vi "#76_MAV_MSG_COMMAND_LONG_ENCODE.vi"(10 "packet_sequence_in":u8, 11 "COMMAND_LONG":T1={"self"={"system_id"=255, "component_id"=190}, "target_system"=1, "target_component"=1, "command (MAV_CMD)"=0, "confirmation"=0, "param1"=0.0, "param2"=0.0, "param3"=0.0, "param4"=0.0, "param5"=0.0, "param6"=0.0, "param7"=0.0}) -> (2 "packet_sequence_out":u8, 3 "mavlink_buffer_out":u8[](array[numeric]))   [LabVIEW 2023]
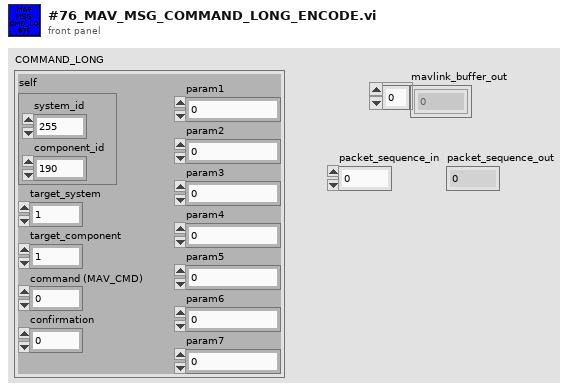
[diagram p1: front panel]
types:
  T1 = cluster{"self":cluster{"system_id":u8, "component_id":u8}, "target_system":u8, "target_component":u8, "command (MAV_CMD)":u16, "confirmation":u8, "param1":sgl, "param2":sgl, "param3":sgl, "param4":sgl, "param5":sgl, "param6":sgl, "param7":sgl}
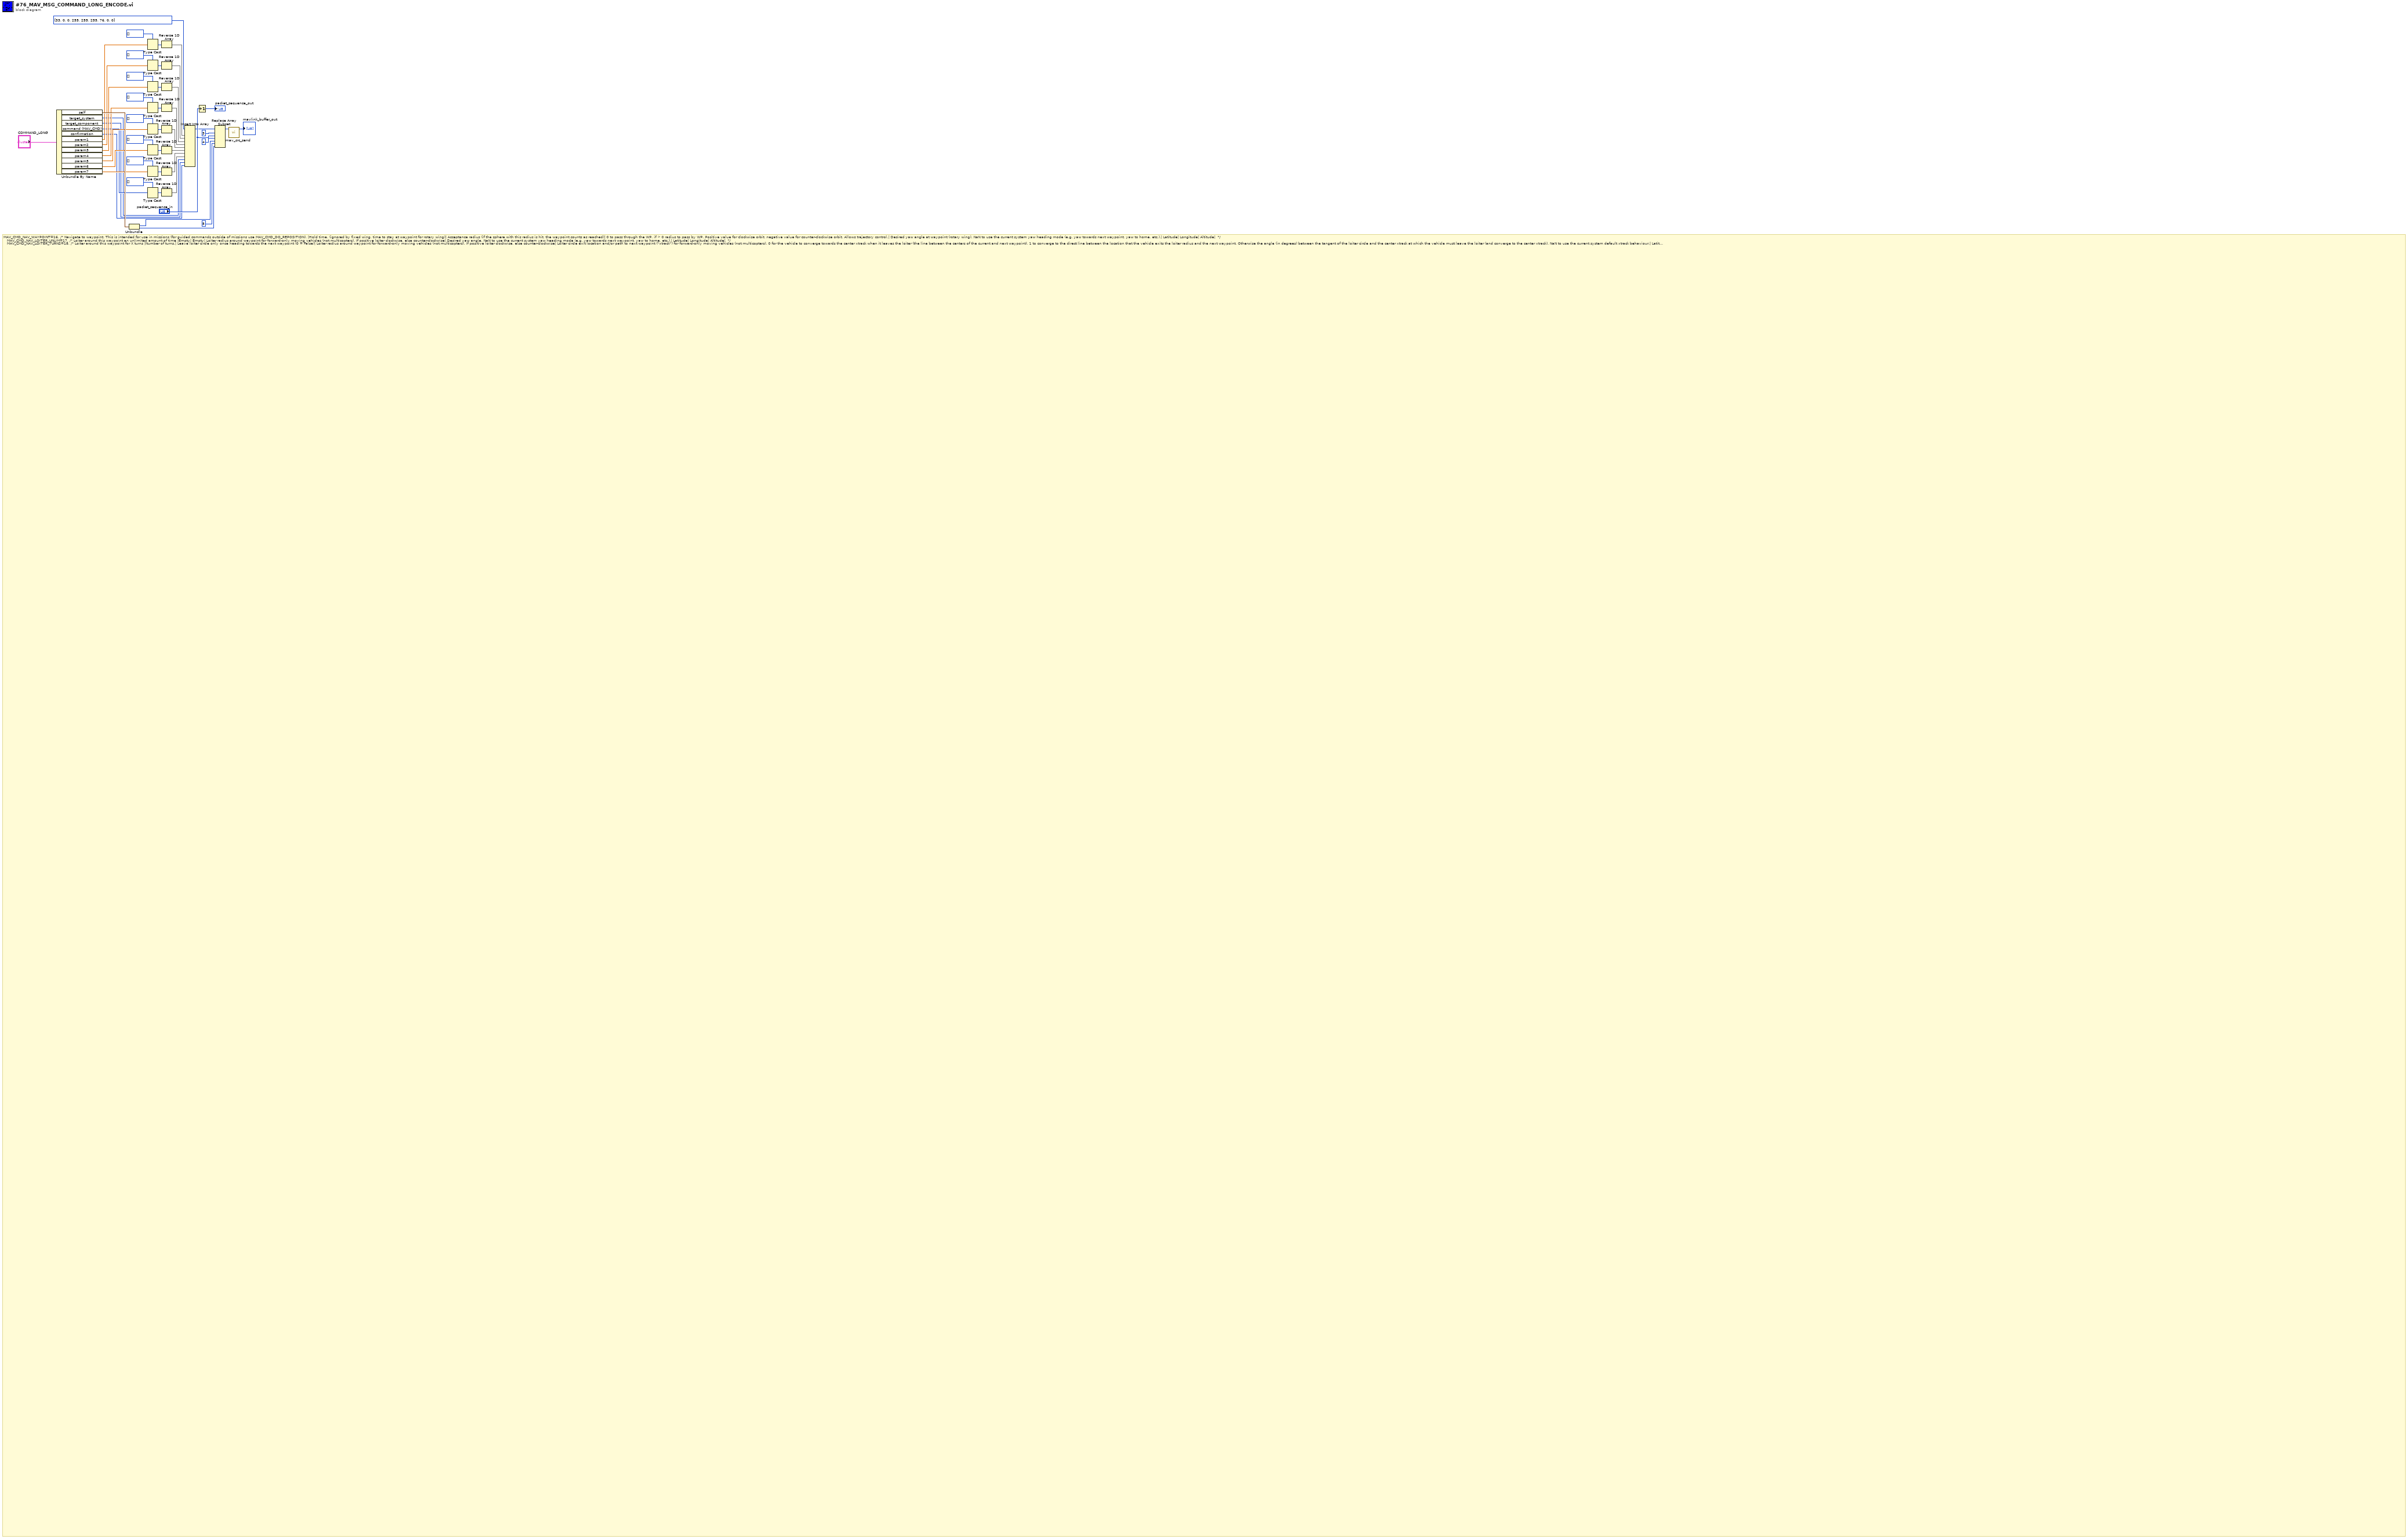
[diagram p0: block diagram]
diagram:
  # "MAV_CMD_NAV_WAYPOINT=16, /* Navigate to waypoint. This is intended for use in missions (for guided commands outside of missions use MAV_CMD_DO_REPOSITION). |Hold time. (ignored by fixed wing, time to stay at waypoint for rotary wing)| Acceptance radius (if the sphere with this radius is hit, the waypoint counts as reached)| 0 to pass through the WP, if > 0 radius to pass by WP. Positive value for clockwise orbit, negative value for counter-clockwise orbit. Allows trajectory control.| Desired yaw angle at waypoint (rotary wing). NaN to use the current system yaw heading mode (e.g. yaw towards next waypoint, yaw to home, etc.).| Latitude| Longitude| Altitude|  */\n   MAV_CMD_NAV_LOITER_UNLIM=17, /* Loiter around this waypoint an unlimited amount of time |Empty| Empty| Loiter radius around waypoint for forward-only moving vehicles (not multicopters). If positive loiter clockwise, else counter-clockwise| Desired yaw angle. NaN to use the current system yaw heading mode (e.g. yaw towards next waypoint, yaw to home, etc.).| Latitude| Longitude| Altitude|  */\n   MAV_CMD_NAV_LOITER_TURNS=18, /* Loiter around this waypoint for X turns |Number of turns.| Leave loiter circle only once heading towards the next waypoint (0 = False)| Loiter radius around waypoint for forward-only moving vehicles (not multicopters). If positive loiter clockwise, else counter-clockwise| Loiter circle exit location and/or path to next waypoint (\"xtrack\") for forward-only moving vehicles (not multicopters). 0 for the vehicle to converge towards the center xtrack when it leaves the loiter (the line between the centers of the current and next waypoint), 1 to converge to the direct line between the location that the vehicle exits the loiter radius and the next waypoint. Otherwise the angle (in degrees) between the tangent of the loiter circle and the center xtrack at which the vehicle must leave the loiter (and converge to the center xtrack). NaN to use the current system default xtrack behaviour.| Latitude| Longitude| Altitude|  */\n   MAV_CMD_NAV_LOITER_TIME=19, /* Loiter at the specified latitude, longitude and altitude for a certain amount of time. Multicopter vehicles stop at the point (within a vehicle-specific acceptance radius). Forward-only moving vehicles (e.g. fixed-wing) circle the point with the specified radius/direction. If the Heading Required parameter (2) is non-zero forward moving aircraft will only leave the loiter circle once heading towards the next waypoint. |Loiter time (only starts once Lat, Lon and Alt is reached).| Leave loiter circle only once heading towards the next waypoint (0 = False)| Loiter radius around waypoint for forward-only moving vehicles (not multicopters). If positive loiter clockwise, else counter-clockwise.| Loiter circle exit location and/or path to next waypoint (\"xtrack\") for forward-only moving vehicles (not multicopters). 0 for the vehicle to converge towards the center xtrack when it leaves the loiter (the line between the centers of the current and next waypoint), 1 to converge to the direct line between the location that the vehicle exits the loiter radius and the next waypoint. Otherwise the angle (in degrees) between the tangent of the loiter circle and the center xtrack at which the vehicle must leave the loiter (and converge to the center xtrack). NaN to use the current system default xtrack behaviour.| Latitude| Longitude| Altitude|  */\n   MAV_CMD_NAV_RETURN_TO_LAUNCH=20, /* Return to launch location |Empty| Empty| Empty| Empty| Empty| Empty| Empty|  */\n   MAV_CMD_NAV_LAND=21, /* Land at location. |Minimum target altitude if landing is aborted (0 = undefined/use system default).| Precision land mode.| Empty.| Desired yaw angle. NaN to use the current system yaw heading mode (e.g. yaw towards next waypoint, yaw to home, etc.).| Latitude.| Longitude.| Landing altitude (ground level in current frame).|  */\n   MAV_CMD_NAV_TAKEOFF=22, /* Takeoff from ground / hand. Vehicles that support multiple takeoff modes (e.g. VTOL quadplane) should take off using the currently configured mode. |Minimum pitch (if airspeed sensor present), desired pitch without sensor| Empty| Empty| Yaw angle (if magnetometer present), ignored without magnetometer. NaN to use the current system yaw heading mode (e.g. yaw towards next waypoint, yaw to home, etc.).| Latitude| Longitude| Altitude|  */\n   MAV_CMD_NAV_LAND_LOCAL=23, /* Land at local position (local frame only) |Landing target number (if available)| Maximum accepted offset from desired landing position - computed magnitude from spherical coordinates: d = sqrt(x^2 + y^2 + z^2), which gives the maximum accepted distance between the desired landing position and the position where the vehicle is about to land| Landing descend rate| Desired yaw angle| Y-axis position| X-axis position| Z-axis / ground level position|  */\n   MAV_CMD_NAV_TAKEOFF_LOCAL=24, /* Takeoff from local position (local frame only) |Minimum pitch (if airspeed sensor present), desired pitch without sensor| Empty| Takeoff ascend rate| Yaw angle (if magnetometer or another yaw estimation source present), ignored without one of these| Y-axis position| X-axis position| Z-axis position|  */\n   MAV_CMD_NAV_FOLLOW=25, /* Vehicle following, i.e. this waypoint represents the position of a moving vehicle |Following logic to use (e.g. loitering or sinusoidal following) - depends on specific autopilot implementation| Ground speed of vehicle to be followed| Radius around waypoint. If positive loiter clockwise, else counter-clockwise| Desired yaw angle.| Latitude| Longitude| Altitude|  */\n   MAV_CMD_NAV_CONTINUE_AND_CHANGE_ALT=30, /* Continue on the current course and climb/descend to specified altitude.  When the altitude is reached continue to the next command (i.e., don't proceed to the next command until the desired altitude is reached. |Climb or Descend (0 = Neutral, command completes when within 5m of this command's altitude, 1 = Climbing, command completes when at or above this command's altitude, 2 = Descending, command completes when at or below this command's altitude.| Empty| Empty| Empty| Empty| Empty| Desired altitude|  */\n   MAV_CMD_NAV_LOITER_TO_ALT=31, /* Begin loiter at the specified Latitude and Longitude.  If Lat=Lon=0, then loiter at the current position.  Don't consider the navigation command complete (don't leave loiter) until the altitude has been reached. Additionally, if the Heading Required parameter is non-zero the aircraft will not leave the loiter until heading toward the next waypoint. |Leave loiter circle only once heading towards the next waypoint (0 = False)| Loiter radius around waypoint for forward-only moving vehicles (not multicopters). If positive loiter clockwise, negative counter-clockwise, 0 means no change to standard loiter.| Empty| Loiter circle exit location and/or path to next waypoint (\"xtrack\") for forward-only moving vehicles (not multicopters). 0 for the vehicle to converge towards the center xtrack when it leaves the loiter (the line between the centers of the current and next waypoint), 1 to converge to the direct line between the location that the vehicle exits the loiter radius and the next waypoint. Otherwise the angle (in degrees) between the tangent of the loiter circle and the center xtrack at which the vehicle must leave the loiter (and converge to the center xtrack). NaN to use the current system default xtrack behaviour.| Latitude| Longitude| Altitude|  */\n   MAV_CMD_DO_FOLLOW=32, /* Begin following a target |System ID (of the FOLLOW_TARGET beacon). Send 0 to disable follow-me and return to the default position hold mode.| Reserved| Reserved| Altitude mode: 0: Keep current altitude, 1: keep altitude difference to target, 2: go to a fixed altitude above home.| Altitude above home. (used if mode=2)| Reserved| Time to land in which the MAV should go to the default position hold mode after a message RX timeout.|  */\n   MAV_CMD_DO_FOLLOW_REPOSITION=33, /* Reposition the MAV after a follow target command has been sent |Camera q1 (where 0 is on the ray from the camera to the tracking device)| Camera q2| Camera q3| Camera q4| altitude offset from target| X offset from target| Y offset from target|  */\n   MAV_CMD_DO_ORBIT=34, /* Start orbiting on the circumference of a circle defined by the parameters. Setting values to NaN/INT32_MAX (as appropriate) results in using defaults. |Radius of the circle. Positive: orbit clockwise. Negative: orbit counter-clockwise. NaN: Use vehicle default radius, or current radius if already orbiting.| Tangential Velocity. NaN: Use vehicle default velocity, or current velocity if already orbiting.| Yaw behavior of the vehicle.| Orbit around the centre point for this many radians (i.e. for a three-quarter orbit set 270*Pi/180). 0: Orbit forever. NaN: Use vehicle default, or current value if already orbiting.| Center point latitude (if no MAV_FRAME specified) / X coordinate according to MAV_FRAME. INT32_MAX (or NaN if sent in COMMAND_LONG): Use current vehicle position, or current center if already orbiting.| Center point longitude (if no MAV_FRAME specified) / Y coordinate according to MAV_FRAME. INT32_MAX (or NaN if sent in COMMAND_LONG): Use current vehicle position, or current center if already orbiting.| Center point altitude (MSL) (if no MAV_FRAME specified) / Z coordinate according to MAV_FRAME. NaN: Use current vehicle altitude.|  */\n   MAV_CMD_NAV_ROI=80, /* Sets the region of interest (ROI) for a sensor set or the vehicle itself. This can then be used by the vehicle's control system to control the vehicle attitude and the attitude of various sensors such as cameras. |Region of interest mode.| Waypoint index/ target ID. (see MAV_ROI enum)| ROI index (allows a vehicle to manage multiple ROI's)| Empty| x the location of the fixed ROI (see MAV_FRAME)| y| z|  */\n   MAV_CMD_NAV_PATHPLANNING=81, /* Control autonomous path planning on the MAV. |0: Disable local obstacle avoidance / local path planning (without resetting map), 1: Enable local path planning, 2: Enable and reset local path planning| 0: Disable full path planning (without resetting map), 1: Enable, 2: Enable and reset map/occupancy grid, 3: Enable and reset planned route, but not occupancy grid| Empty| Yaw angle at goal| Latitude/X of goal| Longitude/Y of goal| Altitude/Z of goal|  */\n   MAV_CMD_NAV_SPLINE_WAYPOINT=82, /* Navigate to waypoint using a spline path. |Hold time. (ignored by fixed wing, time to stay at waypoint for rotary wing)| Empty| Empty| Empty| Latitude/X of goal| Longitude/Y of goal| Altitude/Z of goal|  */\n   MAV_CMD_NAV_VTOL_TAKEOFF=84, /* Takeoff from ground using VTOL mode, and transition to forward flight with specified heading. The command should be ignored by vehicles that dont support both VTOL and fixed-wing flight (multicopters, boats,etc.). |Empty| Front transition heading.| Empty| Yaw angle. NaN to use the current system yaw heading mode (e.g. yaw towards next waypoint, yaw to home, etc.).| Latitude| Longitude| Altitude|  */\n   MAV_CMD_NAV_VTOL_LAND=85, /* Land using VTOL mode |Landing behaviour.| Empty| Approach altitude (with the same reference as the Altitude field). NaN if unspecified.| Yaw angle. NaN to use the current system yaw heading mode (e.g. yaw towards next waypoint, yaw to home, etc.).| Latitude| Longitude| Altitude (ground level) relative to the current coordinate frame. NaN to use system default landing altitude (ignore value).|  */\n   MAV_CMD_NAV_GUIDED_ENABLE=92, /* hand control over to an external controller |On / Off (> 0.5f on)| Empty| Empty| Empty| Empty| Empty| Empty|  */\n   MAV_CMD_NAV_DELAY=93, /* Delay the next navigation command a number of seconds or until a specified time |Delay (-1 to enable time-of-day fields)| hour (24h format, UTC, -1 to ignore)| minute (24h format, UTC, -1 to ignore)| second (24h format, UTC, -1 to ignore)| Empty| Empty| Empty|  */\n   MAV_CMD_NAV_PAYLOAD_PLACE=94, /* Descend and place payload. Vehicle moves to specified location, descends until it detects a hanging payload has reached the ground, and then releases the payload. If ground is not detected before the reaching the maximum descent value (param1), the command will complete without releasing the payload. |Maximum distance to descend.| Empty| Empty| Empty| Latitude| Longitude| Altitude|  */\n   MAV_CMD_NAV_LAST=95, /* NOP - This command is only used to mark the upper limit of the NAV/ACTION commands in the enumeration |Empty| Empty| Empty| Empty| Empty| Empty| Empty|  */\n   MAV_CMD_CONDITION_DELAY=112, /* Delay mission state machine. |Delay| Empty| Empty| Empty| Empty| Empty| Empty|  */\n   MAV_CMD_CONDITION_CHANGE_ALT=113, /* Ascend/descend to target altitude at specified rate. Delay mission state machine until desired altitude reached. |Descent / Ascend rate.| Empty| Empty| Empty| Empty| Empty| Target Altitude|  */\n   MAV_CMD_CONDITION_DISTANCE=114, /* Delay mission state machine until within desired distance of next NAV point. |Distance.| Empty| Empty| Empty| Empty| Empty| Empty|  */\n   MAV_CMD_CONDITION_YAW=115, /* Reach a certain target angle. |target angle [0-360]. Absolute angles: 0 is north. Relative angle: 0 is initial yaw. Direction set by param3.| angular speed| direction: -1: counter clockwise, 0: shortest direction, 1: clockwise| 0: absolute angle, 1: relative offset| Empty| Empty| Empty|  */\n   MAV_CMD_CONDITION_LAST=159, /* NOP - This command is only used to mark the upper limit of the CONDITION commands in the enumeration |Empty| Empty| Empty| Empty| Empty| Empty| Empty|  */\n   MAV_CMD_DO_SET_MODE=176, /* Set system mode. |Mode| Custom mode - this is system specific, please refer to the individual autopilot specifications for details.| Custom sub mode - this is system specific, please refer to the individual autopilot specifications for details.| Empty| Empty| Empty| Empty|  */\n   MAV_CMD_DO_JUMP=177, /* Jump to the desired command in the mission list.  Repeat this action only the specified number of times |Sequence number| Repeat count| Empty| Empty| Empty| Empty| Empty|  */\n   MAV_CMD_DO_CHANGE_SPEED=178, /* Change speed and/or throttle set points. The value persists until it is overridden or there is a mode change |Speed type of value set in param2 (such as airspeed, ground speed, and so on)| Speed (-1 indicates no change, -2 indicates return to default vehicle speed)| Throttle (-1 indicates no change, -2 indicates return to default vehicle throttle value)| Reserved (default:0)| Reserved (default:0)| Reserved (default:0)| Reserved (default:0)|  */\n   MAV_CMD_DO_SET_HOME=179, /* \n          Sets the home position to either to the current position or a specified position.\n          The home position is the default position that the system will return to and land on.\n          The position is set automatically by the system during the takeoff (and may also be set using this command).\n          Note: the current home position may be emitted in a HOME_POSITION message on request (using MAV_CMD_REQUEST_MESSAGE with param1=242).\n         |Use current (1=use current location, 0=use specified location)| Roll angle (of surface). Range: -180..180 degrees. NAN or 0 means value not set. 0.01 indicates zero roll.| Pitch angle (of surface). Range: -90..90 degrees. NAN or 0 means value not set. 0.01 means zero pitch.| Yaw angle. NaN to use default heading. Range: -180..180 degrees.| Latitude| Longitude| Altitude|  */\n   MAV_CMD_DO_SET_PARAMETER=180, /* Set a system parameter.  Caution!  Use of this command requires knowledge of the numeric enumeration value of the parameter. |Parameter number| Parameter value| Empty| Empty| Empty| Empty| Empty|  */\n   MAV_CMD_DO_SET_RELAY=181, /* Set a relay to a condition. |Relay instance number.| Setting. (1=on, 0=off, others possible depending on system hardware)| Empty| Empty| Empty| Empty| Empty|  */\n   MAV_CMD_DO_REPEAT_RELAY=182, /* Cycle a relay on and off for a desired number of cycles with a desired period. |Relay instance number.| Cycle count.| Cycle time.| Empty| Empty| Empty| Empty|  */\n   MAV_CMD_DO_SET_SERVO=183, /* Set a servo to a desired PWM value. |Servo instance number.| Pulse Width Modulation.| Empty| Empty| Empty| Empty| Empty|  */\n   MAV_CMD_DO_REPEAT_SERVO=184, /* Cycle a between its nominal setting and a desired PWM for a desired number of cycles with a desired period. |Servo instance number.| Pulse Width Modulation.| Cycle count.| Cycle time.| Empty| Empty| Empty|  */\n   MAV_CMD_DO_FLIGHTTERMINATION=185, /* Terminate flight immediately.\n          Flight termination immediately and irreversibly terminates the current flight, returning the vehicle to ground.\n          The vehicle will ignore RC or other input until it has been power-cycled.\n          Termination may trigger safety measures, including: disabling motors and deployment of parachute on multicopters, and setting flight surfaces to initiate a landing pattern on fixed-wing).\n          On multicopters without a parachute it may trigger a crash landing.\n          Support for this command can be tested using the protocol bit: MAV_PROTOCOL_CAPABILITY_FLIGHT_TERMINATION.\n          Support for this command can also be tested by sending the command with param1=0 (< 0.5); the ACK should be either MAV_RESULT_FAILED or MAV_RESULT_UNSUPPORTED.\n         |Flight termination activated if > 0.5. Otherwise not activated and ACK with MAV_RESULT_FAILED.| Empty| Empty| Empty| Empty| Empty| Empty|  */\n   MAV_CMD_DO_CHANGE_ALTITUDE=186, /* Change altitude set point. |Altitude.| Frame of new altitude.| Empty| Empty| Empty| Empty| Empty|  */\n   MAV_CMD_DO_SET_ACTUATOR=187, /* Sets actuators (e.g. servos) to a desired value. The actuator numbers are mapped to specific outputs (e.g. on any MAIN or AUX PWM or UAVCAN) using a flight-stack specific mechanism (i.e. a parameter). |Actuator 1 value, scaled from [-1 to 1]. NaN to ignore.| Actuator 2 value, scaled from [-1 to 1]. NaN to ignore.| Actuator 3 value, scaled from [-1 to 1]. NaN to ignore.| Actuator 4 value, scaled from [-1 to 1]. NaN to ignore.| Actuator 5 value, scaled from [-1 to 1]. NaN to ignore.| Actuator 6 value, scaled from [-1 to 1]. NaN to ignore.| Index of actuator set (i.e if set to 1, Actuator 1 becomes Actuator 7)|  */\n   MAV_CMD_DO_RETURN_PATH_START=188, /* Mission item to specify the start of a failsafe/landing return-path segment (the end of the segment is the next MAV_CMD_DO_LAND_START item).\n          A vehicle that is using missions for landing (e.g. in a return mode) will join the mission on the closest path of the return-path segment (instead of MAV_CMD_DO_LAND_START or the nearest waypoint).\n          The main use case is to minimize the failsafe flight path in corridor missions, where the inbound/outbound paths are constrained (by geofences) to the same particular path.\n          The MAV_CMD_NAV_RETURN_PATH_START would be placed at the start of the return path.\n          If a failsafe occurs on the outbound path the vehicle will move to the nearest point on the return path (which is parallel for this kind of mission), effectively turning round and following the shortest path to landing.\n          If a failsafe occurs on the inbound path the vehicle is already on the return segment and will continue to landing.\n          The Latitude/Longitude/Altitude are optional, and may be set to 0 if not needed.\n          If specified, the item defines the waypoint at which the return segment starts.\n          If sent using as a command, the vehicle will perform a mission landing (using the land segment if defined) or reject the command if mission landings are not supported, or no mission landing is defined. When used as a command any position information in the command is ignored.\n         |Empty| Empty| Empty| Empty| Latitudee. 0: not used.| Longitudee. 0: not used.| Altitudee. 0: not used.|  */\n   MAV_CMD_DO_LAND_START=189, /* Mission command to perform a landing. This is used as a marker in a mission to tell the autopilot where a sequence of mission items that represents a landing starts.\n\t  It may also be sent via a COMMAND_LONG to trigger a landing, in which case the nearest (geographically) landing sequence in the mission will be used.\n\t  The Latitude/Longitude/Altitude is optional, and may be set to 0 if not needed. If specified then it will be used to help find the closest landing sequence.\n\t |Empty| Empty| Empty| Empty| Latitude| Longitude| Altitude|  */\n   MAV_CMD_DO_RALLY_LAND=190, /* Mission command to perform a landing from a rally point. |Break altitude| Landing speed| Empty| Empty| Empty| Empty| Empty|  */\n   MAV_CMD_DO_GO_AROUND=191, /* Mission command to safely abort an autonomous landing. |Altitude| Empty| Empty| Empty| Empty| Empty| Empty|  */\n   MAV_CMD_DO_REPOSITION=192, /* Reposition the vehicle to a specific WGS84 global position. This command is intended for guided commands (for missions use MAV_CMD_NAV_WAYPOINT instead). |Ground speed, less than 0 (-1) for default| Bitmask of option flags.| Loiter radius for planes. Positive values only, direction is controlled by Yaw value. A value of zero or NaN is ignored. | Yaw heading. NaN to use the current system yaw heading mode (e.g. yaw towards next waypoint, yaw to home, etc.). For planes indicates loiter direction (0: clockwise, 1: counter clockwise)| Latitude| Longitude| Altitude|  */\n   MAV_CMD_DO_PAUSE_CONTINUE=193, /* If in a GPS controlled position mode, hold the current position or continue. |0: Pause current mission or reposition command, hold current position. 1: Continue mission. A VTOL capable vehicle should enter hover mode (multicopter and VTOL planes). A plane should loiter with the default loiter radius.| Reserved| Reserved| Reserved| Reserved| Reserved| Reserved|  */\n   MAV_CMD_DO_SET_REVERSE=194, /* Set moving direction to forward or reverse. |Direction (0=Forward, 1=Reverse)| Empty| Empty| Empty| Empty| Empty| Empty|  */\n   MAV_CMD_DO_SET_ROI_LOCATION=195, /* Sets the region of interest (ROI) to a location. This can then be used by the vehicle's control system to control the vehicle attitude and the attitude of various sensors such as cameras. This command can be sent to a gimbal manager but not to a gimbal device. A gimbal is not to react to this message. |Component ID of gimbal device to address (or 1-6 for non-MAVLink gimbal), 0 for all gimbal device components. Send command multiple times for more than one gimbal (but not all gimbals).| Empty| Empty| Empty| Latitude of ROI location| Longitude of ROI location| Altitude of ROI location|  */\n   MAV_CMD_DO_SET_ROI_WPNEXT_OFFSET=196, /* Sets the region of interest (ROI) to be toward next waypoint, with optional pitch/roll/yaw offset. This can then be used by the vehicle's control system to control the vehicle attitude and the attitude of various sensors such as cameras. This command can be sent to a gimbal manager but not to a gimbal device. A gimbal device is not to react to this message. |Component ID of gimbal device to address (or 1-6 for non-MAVLink gimbal), 0 for all gimbal device components. Send command multiple times for more than one gimbal (but not all gimbals).| Empty| Empty| Empty| Pitch offset from next waypoint, positive pitching up| Roll offset from next waypoint, positive rolling to the right| Yaw offset from next waypoint, positive yawing to the right|  */\n   MAV_CMD_DO_SET_ROI_NONE=197, /* Cancels any previous ROI command returning the vehicle/sensors to default flight characteristics. This can then be used by the vehicle's control system to control the vehicle attitude and the attitude of various sensors such as cameras. This command can be sent to a gimbal manager but not to a gimbal device. A gimbal device is not to react to this message. After this command the gimbal manager should go back to manual input if available, and otherwise assume a neutral position. |Component ID of gimbal device to address (or 1-6 for non-MAVLink gimbal), 0 for all gimbal device components. Send command multiple times for more than one gimbal (but not all gimbals).| Empty| Empty| Empty| Empty| Empty| Empty|  */\n   MAV_CMD_DO_SET_ROI_SYSID=198, /* Mount tracks system with specified system ID. Determination of target vehicle position may be done with GLOBAL_POSITION_INT or any other means. This command can be sent to a gimbal manager but not to a gimbal device. A gimbal device is not to react to this message. |System ID| Component ID of gimbal device to address (or 1-6 for non-MAVLink gimbal), 0 for all gimbal device components. Send command multiple times for more than one gimbal (but not all gimbals).| Reserved (default:0)| Reserved (default:0)| Reserved (default:0)| Reserved (default:0)| Reserved (default:0)|  */\n   MAV_CMD_DO_CONTROL_VIDEO=200, /* Control onboard camera system. |Camera ID (-1 for all)| Transmission: 0: disabled, 1: enabled compressed, 2: enabled raw| Transmission mode: 0: video stream, >0: single images every n seconds| Recording: 0: disabled, 1: enabled compressed, 2: enabled raw| Empty| Empty| Empty|  */\n   MAV_CMD_DO_SET_ROI=201, /* Sets the region of interest (ROI) for a sensor set or the vehicle itself. This can then be used by the vehicle's control system to control the vehicle attitude and the attitude of various sensors such as cameras. |Region of interest mode.| Waypoint index/ target ID (depends on param 1).| Region of interest index. (allows a vehicle to manage multiple ROI's)| Empty| MAV_ROI_WPNEXT: pitch offset from next waypoint, MAV_ROI_LOCATION: latitude| MAV_ROI_WPNEXT: roll offset from next waypoint, MAV_ROI_LOCATION: longitude| MAV_ROI_WPNEXT: yaw offset from next waypoint, MAV_ROI_LOCATION: altitude|  */\n   MAV_CMD_DO_DIGICAM_CONFIGURE=202, /* Configure digital camera. This is a fallback message for systems that have not yet implemented PARAM_EXT_XXX messages and camera definition files (see https://mavlink.io/en/services/camera_def.html ). |Modes: P, TV, AV, M, Etc.| Shutter speed: Divisor number for one second.| Aperture: F stop number.| ISO number e.g. 80, 100, 200, Etc.| Exposure type enumerator.| Command Identity.| Main engine cut-off time before camera trigger. (0 means no cut-off)|  */\n   MAV_CMD_DO_DIGICAM_CONTROL=203, /* Control digital camera. This is a fallback message for systems that have not yet implemented PARAM_EXT_XXX messages and camera definition files (see https://mavlink.io/en/services/camera_def.html ). |Session control e.g. show/hide lens| Zoom's absolute position| Zooming step value to offset zoom from the current position| Focus Locking, Unlocking or Re-locking| Shooting Command| Command Identity| Test shot identifier. If set to 1, image will only be captured, but not counted towards internal frame count.|  */\n   MAV_CMD_DO_MOUNT_CONFIGURE=204, /* Mission command to configure a camera or antenna mount |Mount operation mode| stabilize roll? (1 = yes, 0 = no)| stabilize pitch? (1 = yes, 0 = no)| stabilize yaw? (1 = yes, 0 = no)| roll input (0 = angle body frame, 1 = angular rate, 2 = angle absolute frame)| pitch input (0 = angle body frame, 1 = angular rate, 2 = angle absolute frame)| yaw input (0 = angle body frame, 1 = angular rate, 2 = angle absolute frame)|  */\n   MAV_CMD_DO_MOUNT_CONTROL=205, /* Mission command to control a camera or antenna mount |pitch depending on mount mode (degrees or degrees/second depending on pitch input).| roll depending on mount mode (degrees or degrees/second depending on roll input).| yaw depending on mount mode (degrees or degrees/second depending on yaw input).| altitude depending on mount mode.| latitude, set if appropriate mount mode.| longitude, set if appropriate mount mode.| Mount mode.|  */\n   MAV_CMD_DO_SET_CAM_TRIGG_DIST=206, /* Mission command to set camera trigger distance for this flight. The camera is triggered each time this distance is exceeded. This command can also be used to set the shutter integration time for the camera. |Camera trigger distance. 0 to stop triggering.| Camera shutter integration time. -1 or 0 to ignore| Trigger camera once immediately. (0 = no trigger, 1 = trigger)| Empty| Empty| Empty| Empty|  */\n   MAV_CMD_DO_FENCE_ENABLE=207, /* \n          Enable the geofence.\n          This can be used in a mission or via the command protocol.\n          The persistence/lifetime of the setting is undefined.\n          Depending on flight stack implementation it may persist until superseded, or it may revert to a system default at the end of a mission.\n          Flight stacks typically reset the setting to system defaults on reboot.\n\t |enable? (0=disable, 1=enable, 2=disable_floor_only)| Fence types to enable or disable as a bitmask. A value of 0 indicates that all fences should be enabled or disabled. This parameter is ignored if param 1 has the value 2| Empty| Empty| Empty| Empty| Empty|  */\n   MAV_CMD_DO_PARACHUTE=208, /* Mission item/command to release a parachute or enable/disable auto release. |Action| Empty| Empty| Empty| Empty| Empty| Empty|  */\n   MAV_CMD_DO_MOTOR_TEST=209, /* Command to perform motor test. |Motor instance number (from 1 to max number of motors on the vehicle).| Throttle type (whether the Throttle Value in param3 is a percentage, PWM value, etc.)| Throttle value.| Timeout between tests that are run in sequence.| Motor count. Number of motors to test in sequence: 0/1=one motor, 2= two motors, etc. The Timeout (param4) is used between tests.| Motor test order.| Empty|  */\n   MAV_CMD_DO_INVERTED_FLIGHT=210, /* Change to/from inverted flight. |Inverted flight. (0=normal, 1=inverted)| Empty| Empty| Empty| Empty| Empty| Empty|  */\n   MAV_CMD_DO_GRIPPER=211, /* Mission command to operate a gripper. |Gripper instance number.| Gripper action to perform.| Empty| Empty| Empty| Empty| Empty|  */\n   MAV_CMD_DO_AUTOTUNE_ENABLE=212, /* Enable/disable autotune. |Enable (1: enable, 0:disable).| Specify which axis are autotuned. 0 indicates autopilot default settings.| Empty.| Empty.| Empty.| Empty.| Empty.|  */\n   MAV_CMD_NAV_SET_YAW_SPEED=213, /* Sets a desired vehicle turn angle and speed change. |Yaw angle to adjust steering by.| Speed.| Final angle. (0=absolute, 1=relative)| Empty| Empty| Empty| Empty|  */\n   MAV_CMD_DO_SET_CAM_TRIGG_INTERVAL=214, /* Mission command to set camera trigger interval for this flight. If triggering is enabled, the camera is triggered each time this interval expires. This command can also be used to set the shutter integration time for the camera. |Camera trigger cycle time. -1 or 0 to ignore.| Camera shutter integration time. Should be less than trigger cycle time. -1 or 0 to ignore.| Empty| Empty| Empty| Empty| Empty|  */\n   MAV_CMD_DO_MOUNT_CONTROL_QUAT=220, /* Mission command to control a camera or antenna mount, using a quaternion as reference. |quaternion param q1, w (1 in null-rotation)| quaternion param q2, x (0 in null-rotation)| quaternion param q3, y (0 in null-rotation)| quaternion param q4, z (0 in null-rotation)| Empty| Empty| Empty|  */\n   MAV_CMD_DO_GUIDED_MASTER=221, /* set id of master controller |System ID| Component ID| Empty| Empty| Empty| Empty| Empty|  */\n   MAV_CMD_DO_GUIDED_LIMITS=222, /* Set limits for external control |Timeout - maximum time that external controller will be allowed to control vehicle. 0 means no timeout.| Altitude (MSL) min - if vehicle moves below this alt, the command will be aborted and the mission will continue. 0 means no lower altitude limit.| Altitude (MSL) max - if vehicle moves above this alt, the command will be aborted and the mission will continue. 0 means no upper altitude limit.| Horizontal move limit - if vehicle moves more than this distance from its location at the moment the command was executed, the command will be aborted and the mission will continue. 0 means no horizontal move limit.| Empty| Empty| Empty|  */\n   MAV_CMD_DO_ENGINE_CONTROL=223, /* Control vehicle engine. This is interpreted by the vehicles engine controller to change the target engine state. It is intended for vehicles with internal combustion engines |0: Stop engine, 1:Start Engine| 0: Warm start, 1:Cold start. Controls use of choke where applicable| Height delay. This is for commanding engine start only after the vehicle has gained the specified height. Used in VTOL vehicles during takeoff to start engine after the aircraft is off the ground. Zero for no delay.| Empty| Empty| Empty| Empty|  */\n   MAV_CMD_DO_SET_MISSION_CURRENT=224, /* \n          Set the mission item with sequence number seq as the current item and emit MISSION_CURRENT (whether or not the mission number changed).\n          If a mission is currently being executed, the system will continue to this new mission item on the shortest path, skipping any intermediate mission items.\n\t  Note that mission jump repeat counters are not reset unless param2 is set (see MAV_CMD_DO_JUMP param2).\n\n          This command may trigger a mission state-machine change on some systems: for example from MISSION_STATE_NOT_STARTED or MISSION_STATE_PAUSED to MISSION_STATE_ACTIVE.\n          If the system is in mission mode, on those systems this command might therefore start, restart or resume the mission.\n          If the system is not in mission mode this command must not trigger a switch to mission mode.\n\n          The mission may be \"reset\" using param2.\n          Resetting sets jump counters to initial values (to reset counters without changing the current mission item set the param1 to `-1`).\n          Resetting also explicitly changes a mission state of MISSION_STATE_COMPLETE to MISSION_STATE_PAUSED or MISSION_STATE_ACTIVE, potentially allowing it to resume when it is (next) in a mission mode.\n\n\t  The command will ACK with MAV_RESULT_FAILED if the sequence number is out of range (including if there is no mission item).\n         |Mission sequence value to set. -1 for the current mission item (use to reset mission without changing current mission item).| Resets mission. 1: true, 0: false. Resets jump counters to initial values and changes mission state \"completed\" to be \"active\" or \"paused\".| Empty| Empty| Empty| Empty| Empty|  */\n   MAV_CMD_DO_LAST=240, /* NOP - This command is only used to mark the upper limit of the DO commands in the enumeration |Empty| Empty| Empty| Empty| Empty| Empty| Empty|  */\n   MAV_CMD_PREFLIGHT_CALIBRATION=241, /* Trigger calibration. This command will be only accepted if in pre-flight mode. Except for Temperature Calibration, only one sensor should be set in a single message and all others should be zero. |1: gyro calibration, 3: gyro temperature calibration| 1: magnetometer calibration| 1: ground pressure calibration| 1: radio RC calibration, 2: RC trim calibration| 1: accelerometer calibration, 2: board level calibration, 3: accelerometer temperature calibration, 4: simple accelerometer calibration| 1: APM: compass/motor interference calibration (PX4: airspeed calibration, deprecated), 2: airspeed calibration| 1: ESC calibration, 3: barometer temperature calibration|  */\n   MAV_CMD_PREFLIGHT_SET_SENSOR_OFFSETS=242, /* Set sensor offsets. This command will be only accepted if in pre-flight mode. |Sensor to adjust the offsets for: 0: gyros, 1: accelerometer, 2: magnetometer, 3: barometer, 4: optical flow, 5: second magnetometer, 6: third magnetometer| X axis offset (or generic dimension 1), in the sensor's raw units| Y axis offset (or generic dimension 2), in the sensor's raw units| Z axis offset (or generic dimension 3), in the sensor's raw units| Generic dimension 4, in the sensor's raw units| Generic dimension 5, in the sensor's raw units| Generic dimension 6, in the sensor's raw units|  */\n   MAV_CMD_PREFLIGHT_UAVCAN=243, /* Trigger UAVCAN configuration (actuator ID assignment and direction mapping). Note that this maps to the legacy UAVCAN v0 function UAVCAN_ENUMERATE, which is intended to be executed just once during initial vehicle configuration (it is not a normal pre-flight command and has been poorly named). |1: Trigger actuator ID assignment and direction mapping. 0: Cancel command.| Reserved| Reserved| Reserved| Reserved| Reserved| Reserved|  */\n   MAV_CMD_PREFLIGHT_STORAGE=245, /* Request storage of different parameter values and logs. This command will be only accepted if in pre-flight mode. |Action to perform on the persistent parameter storage| Action to perform on the persistent mission storage| Onboard logging: 0: Ignore, 1: Start default rate logging, -1: Stop logging, > 1: logging rate (e.g. set to 1000 for 1000 Hz logging)| Reserved| Empty| Empty| Empty|  */\n   MAV_CMD_PREFLIGHT_REBOOT_SHUTDOWN=246, /* Request the reboot or shutdown of system components. |0: Do nothing for autopilot, 1: Reboot autopilot, 2: Shutdown autopilot, 3: Reboot autopilot and keep it in the bootloader until upgraded.| 0: Do nothing for onboard computer, 1: Reboot onboard computer, 2: Shutdown onboard computer, 3: Reboot onboard computer and keep it in the bootloader until upgraded.| 0: Do nothing for component, 1: Reboot component, 2: Shutdown component, 3: Reboot component and keep it in the bootloader until upgraded| MAVLink Component ID targeted in param3 (0 for all components).| Reserved (set to 0)| Reserved (set to 0)| WIP: ID (e.g. camera ID -1 for all IDs)|  */\n   MAV_CMD_OVERRIDE_GOTO=252, /* Override current mission with command to pause mission, pause mission and move to position, continue/resume mission. When param 1 indicates that the mission is paused (MAV_GOTO_DO_HOLD), param 2 defines whether it holds in place or moves to another position. |MAV_GOTO_DO_HOLD: pause mission and either hold or move to specified position (depending on param2), MAV_GOTO_DO_CONTINUE: resume mission.| MAV_GOTO_HOLD_AT_CURRENT_POSITION: hold at current position, MAV_GOTO_HOLD_AT_SPECIFIED_POSITION: hold at specified position.| Coordinate frame of hold point.| Desired yaw angle.| Latitude/X position.| Longitude/Y position.| Altitude/Z position.|  */\n   MAV_CMD_OBLIQUE_SURVEY=260, /* Mission command to set a Camera Auto Mount Pivoting Oblique Survey (Replaces CAM_TRIGG_DIST for this purpose). The camera is triggered each time this distance is exceeded, then the mount moves to the next position. Params 4~6 set-up the angle limits and number of positions for oblique survey, where mount-enabled vehicles automatically roll the camera between shots to emulate an oblique camera setup (providing an increased HFOV). This command can also be used to set the shutter integration time for the camera. |Camera trigger distance. 0 to stop triggering.| Camera shutter integration time. 0 to ignore| The minimum interval in which the camera is capable of taking subsequent pictures repeatedly. 0 to ignore.| Total number of roll positions at which the camera will capture photos (images captures spread evenly across the limits defined by param5).| Angle limits that the camera can be rolled to left and right of center.| Fixed pitch angle that the camera will hold in oblique mode if the mount is actuated in the pitch axis.| Empty|  */\n   MAV_CMD_MISSION_START=300, /* start running a mission |first_item: the first mission item to run| last_item:  the last mission item to run (after this item is run, the mission ends)| Reserved (default:0)| Reserved (default:0)| Reserved (default:0)| Reserved (default:0)| Reserved (default:0)|  */\n   MAV_CMD_ACTUATOR_TEST=310, /* Actuator testing command. This is similar to MAV_CMD_DO_MOTOR_TEST but operates on the level of output functions, i.e. it is possible to test Motor1 independent from which output it is configured on. Autopilots typically refuse this command while armed. |Output value: 1 means maximum positive output, 0 to center servos or minimum motor thrust (expected to spin), -1 for maximum negative (if not supported by the motors, i.e. motor is not reversible, smaller than 0 maps to NaN). And NaN maps to disarmed (stop the motors).| Timeout after which the test command expires and the output is restored to the previous value. A timeout has to be set for safety reasons. A timeout of 0 means to restore the previous value immediately.| Reserved (default:0)| Reserved (default:0)| Actuator Output function| Reserved (default:0)| Reserved (default:0)|  */\n   MAV_CMD_CONFIGURE_ACTUATOR=311, /* Actuator configuration command. |Actuator configuration action| Reserved (default:0)| Reserved (default:0)| Reserved (default:0)| Actuator Output function| Reserved (default:0)| Reserved (default:0)|  */\n   MAV_CMD_COMPONENT_ARM_DISARM=400, /* Arms / Disarms a component |0: disarm, 1: arm| 0: arm-disarm unless prevented by safety checks (i.e. when landed), 21196: force arming/disarming (e.g. allow arming to override preflight checks and disarming in flight)| Reserved (default:0)| Reserved (default:0)| Reserved (default:0)| Reserved (default:0)| Reserved (default:0)|  */\n   MAV_CMD_RUN_PREARM_CHECKS=401, /* Instructs a target system to run pre-arm checks.\n          This allows preflight checks to be run on demand, which may be useful on systems that normally run them at low rate, or which do not trigger checks when the armable state might have changed.\n          This command should return MAV_RESULT_ACCEPTED if it will run the checks.\n          The results of the checks are usually then reported in SYS_STATUS messages (this is system-specific).\n          The command should return MAV_RESULT_TEMPORARILY_REJECTED if the system is already armed.\n         |Reserved (default:0)| Reserved (default:0)| Reserved (default:0)| Reserved (default:0)| Reserved (default:0)| Reserved (default:0)| Reserved (default:0)|  */\n   MAV_CMD_ILLUMINATOR_ON_OFF=405, /* Turns illuminators ON/OFF. An illuminator is a light source that is used for lighting up dark areas external to the system: e.g. a torch or searchlight (as opposed to a light source for illuminating the system itself, e.g. an indicator light). |0: Illuminators OFF, 1: Illuminators ON| Reserved (default:0)| Reserved (default:0)| Reserved (default:0)| Reserved (default:0)| Reserved (default:0)| Reserved (default:0)|  */\n   MAV_CMD_DO_ILLUMINATOR_CONFIGURE=406, /* Configures illuminator settings. An illuminator is a light source that is used for lighting up dark areas external to the system: e.g. a torch or searchlight (as opposed to a light source for illuminating the system itself, e.g. an indicator light). |Mode| 0%: Off, 100%: Max Brightness| Strobe period in seconds where 0 means strobing is not used| Strobe duty cycle where 100% means it is on constantly and 0 means strobing is not used| Reserved (default:0)| Reserved (default:0)| Reserved (default:0)|  */\n   MAV_CMD_GET_HOME_POSITION=410, /* Request the home position from the vehicle.\n\t  The vehicle will ACK the command and then emit the HOME_POSITION message. |Reserved| Reserved| Reserved| Reserved| Reserved| Reserved| Reserved|  */\n   MAV_CMD_INJECT_FAILURE=420, /* Inject artificial failure for testing purposes. Note that autopilots should implement an additional protection before accepting this command such as a specific param setting. |The unit which is affected by the failure.| The type how the failure manifests itself.| Instance affected by failure (0 to signal all).| Reserved (default:0)| Reserved (default:0)| Reserved (default:0)| Reserved (default:0)|  */\n   MAV_CMD_START_RX_PAIR=500, /* Starts receiver pairing. |0:Spektrum.| RC type.| Reserved (default:0)| Reserved (default:0)| Reserved (default:0)| Reserved (default:0)| Reserved (default:0)|  */\n   MAV_CMD_GET_MESSAGE_INTERVAL=510, /* \n          Request the interval between messages for a particular MAVLink message ID.\n          The receiver should ACK the command and then emit its response in a MESSAGE_INTERVAL message.\n         |The MAVLink message ID| Reserved (default:0)| Reserved (default:0)| Reserved (default:0)| Reserved (default:0)| Reserved (default:0)| Reserved (default:0)|  */\n   MAV_CMD_SET_MESSAGE_INTERVAL=511, /* Set the interval between messages for a particular MAVLink message ID. This interface replaces REQUEST_DATA_STREAM. |The MAVLink message ID| The interval between two messages. -1: disable. 0: request default rate (which may be zero).| Reserved (default:0)| Reserved (default:0)| Reserved (default:0)| Reserved (default:0)| Target address of message stream (if message has target address fields). 0: Flight-stack default (recommended), 1: address of requestor, 2: broadcast.|  */\n   MAV_CMD_REQUEST_MESSAGE=512, /* Request the target system(s) emit a single instance of a specified message (i.e. a \"one-shot\" version of MAV_CMD_SET_MESSAGE_INTERVAL). |The MAVLink message ID of the requested message.| Use for index ID, if required. Otherwise, the use of this parameter (if any) must be defined in the requested message. By default assumed not used (0).| The use of this parameter (if any), must be defined in the requested message. By default assumed not used (0).| The use of this parameter (if any), must be defined in the requested message. By default assumed not used (0).| The use of this parameter (if any), must be defined in the requested message. By default assumed not used (0).| The use of this parameter (if any), must be defined in the requested message. By default assumed not used (0).| Target address for requested message (if message has target address fields). 0: Flight-stack default, 1: address of requestor, 2: broadcast.|  */\n   MAV_CMD_REQUEST_PROTOCOL_VERSION=519, /* Request MAVLink protocol version compatibility. All receivers should ACK the command and then emit their capabilities in an PROTOCOL_VERSION message |1: Request supported protocol versions by all nodes on the network| Reserved (all remaining params)| Reserved (default:0)| Reserved (default:0)| Reserved (default:0)| Reserved (default:0)| Reserved (default:0)|  */\n   MAV_CMD_REQUEST_AUTOPILOT_CAPABILITIES=520, /* Request autopilot capabilities. The receiver should ACK the command and then emit its capabilities in an AUTOPILOT_VERSION message |1: Request autopilot version| Reserved (all remaining params)| Reserved (default:0)| Reserved (default:0)| Reserved (default:0)| Reserved (default:0)| Reserved (default:0)|  */\n   MAV_CMD_REQUEST_CAMERA_INFORMATION=521, /* Request camera information (CAMERA_INFORMATION). |0: No action 1: Request camera capabilities| Reserved (all remaining params)| Reserved (default:0)| Reserved (default:0)| Reserved (default:0)| Reserved (default:0)| Reserved (default:0)|  */\n   MAV_CMD_REQUEST_CAMERA_SETTINGS=522, /* Request camera settings (CAMERA_SETTINGS). |0: No Action 1: Request camera settings| Reserved (all remaining params)| Reserved (default:0)| Reserved (default:0)| Reserved (default:0)| Reserved (default:0)| Reserved (default:0)|  */\n   MAV_CMD_REQUEST_STORAGE_INFORMATION=525, /* Request storage information (STORAGE_INFORMATION). Use the command's target_component to target a specific component's storage. |Storage ID (0 for all, 1 for first, 2 for second, etc.)| 0: No Action 1: Request storage information| Reserved (all remaining params)| Reserved (default:0)| Reserved (default:0)| Reserved (default:0)| Reserved (default:0)|  */\n   MAV_CMD_STORAGE_FORMAT=526, /* Format a storage medium. Once format is complete, a STORAGE_INFORMATION message is sent. Use the command's target_component to target a specific component's storage. |Storage ID (1 for first, 2 for second, etc.)| Format storage (and reset image log). 0: No action 1: Format storage| Reset Image Log (without formatting storage medium). This will reset CAMERA_CAPTURE_STATUS.image_count and CAMERA_IMAGE_CAPTURED.image_index. 0: No action 1: Reset Image Log| Reserved (all remaining params)| Reserved (default:0)| Reserved (default:0)| Reserved (default:0)|  */\n   MAV_CMD_REQUEST_CAMERA_CAPTURE_STATUS=527, /* Request camera capture status (CAMERA_CAPTURE_STATUS) |0: No Action 1: Request camera capture status| Reserved (all remaining params)| Reserved (default:0)| Reserved (default:0)| Reserved (default:0)| Reserved (default:0)| Reserved (default:0)|  */\n   MAV_CMD_REQUEST_FLIGHT_INFORMATION=528, /* Request flight information (FLIGHT_INFORMATION) |1: Request flight information| Reserved (all remaining params)| Reserved (default:0)| Reserved (default:0)| Reserved (default:0)| Reserved (default:0)| Reserved (default:0)|  */\n   MAV_CMD_RESET_CAMERA_SETTINGS=529, /* Reset all camera settings to Factory Default |0: No Action 1: Reset all settings| Reserved (all remaining params)| Reserved (default:0)| Reserved (default:0)| Reserved (default:0)| Reserved (default:0)| Reserved (default:0)|  */\n   MAV_CMD_SET_CAMERA_MODE=530, /* Set camera running mode. Use NaN for reserved values. GCS will send a MAV_CMD_REQUEST_VIDEO_STREAM_STATUS command after a mode change if the camera supports video streaming. |Reserved (Set to 0)| Camera mode| Reserved (default:NaN)| Reserved (default:NaN)| Reserved (default:0)| Reserved (default:0)| Reserved (default:NaN)|  */\n   MAV_CMD_SET_CAMERA_ZOOM=531, /* Set camera zoom. Camera must respond with a CAMERA_SETTINGS message (on success). |Zoom type| Zoom value. The range of valid values depend on the zoom type.| Reserved (default:NaN)| Reserved (default:NaN)| Reserved (default:0)| Reserved (default:0)| Reserved (default:NaN)|  */\n   MAV_CMD_SET_CAMERA_FOCUS=532, /* Set camera focus. Camera must respond with a CAMERA_SETTINGS message (on success). |Focus type| Focus value| Reserved (default:NaN)| Reserved (default:NaN)| Reserved (default:0)| Reserved (default:0)| Reserved (default:NaN)|  */\n   MAV_CMD_SET_STORAGE_USAGE=533, /* Set that a particular storage is the preferred location for saving photos, videos, and/or other media (e.g. to set that an SD card is used for storing videos).\n          There can only be one preferred save location for each particular media type: setting a media usage flag will clear/reset that same flag if set on any other storage.\n          If no flag is set the system should use its default storage.\n          A target system can choose to always use default storage, in which case it should ACK the command with MAV_RESULT_UNSUPPORTED.\n          A target system can choose to not allow a particular storage to be set as preferred storage, in which case it should ACK the command with MAV_RESULT_DENIED. |Storage ID (1 for first, 2 for second, etc.)| Usage flags| Reserved (default:0)| Reserved (default:0)| Reserved (default:0)| Reserved (default:0)| Reserved (default:0)|  */\n   MAV_CMD_SET_CAMERA_SOURCE=534, /* Set camera source. Changes the camera's active sources on cameras with multiple image sensors. |Component Id of camera to address or 1-6 for non-MAVLink cameras, 0 for all cameras.| Primary Source| Secondary Source. If non-zero the second source will be displayed as picture-in-picture.| Reserved (default:0)| Reserved (default:0)| Reserved (default:0)| Reserved (default:0)|  */\n   MAV_CMD_JUMP_TAG=600, /* Tagged jump target. Can be jumped to with MAV_CMD_DO_JUMP_TAG. |Tag.| Reserved (default:0)| Reserved (default:0)| Reserved (default:0)| Reserved (default:0)| Reserved (default:0)| Reserved (default:0)|  */\n   MAV_CMD_DO_JUMP_TAG=601, /* Jump to the matching tag in the mission list. Repeat this action for the specified number of times. A mission should contain a single matching tag for each jump. If this is not the case then a jump to a missing tag should complete the mission, and a jump where there are multiple matching tags should always select the one with the lowest mission sequence number. |Target tag to jump to.| Repeat count.| Reserved (default:0)| Reserved (default:0)| Reserved (default:0)| Reserved (default:0)| Reserved (default:0)|  */\n   MAV_CMD_DO_GIMBAL_MANAGER_PITCHYAW=1000, /* Set gimbal manager pitch/yaw setpoints (low rate command). It is possible to set combinations of the values below. E.g. an angle as well as a desired angular rate can be used to get to this angle at a certain angular rate, or an angular rate only will result in continuous turning. NaN is to be used to signal unset. Note: only the gimbal manager will react to this command - it will be ignored by a gimbal device. Use GIMBAL_MANAGER_SET_PITCHYAW if you need to stream pitch/yaw setpoints at higher rate.  |Pitch angle (positive to pitch up, relative to vehicle for FOLLOW mode, relative to world horizon for LOCK mode).| Yaw angle (positive to yaw to the right, relative to vehicle for FOLLOW mode, absolute to North for LOCK mode).| Pitch rate (positive to pitch up).| Yaw rate (positive to yaw to the right).| Gimbal manager flags to use.| Reserved (default:0)| Component ID of gimbal device to address (or 1-6 for non-MAVLink gimbal), 0 for all gimbal device components. Send command multiple times for more than one gimbal (but not all gimbals).|  */\n   MAV_CMD_DO_GIMBAL_MANAGER_CONFIGURE=1001, /* Gimbal configuration to set which sysid/compid is in primary and secondary control. |Sysid for primary control (0: no one in control, -1: leave unchanged, -2: set itself in control (for missions where the own sysid is still unknown), -3: remove control if currently in control).| Compid for primary control (0: no one in control, -1: leave unchanged, -2: set itself in control (for missions where the own sysid is still unknown), -3: remove control if currently in control).| Sysid for secondary control (0: no one in control, -1: leave unchanged, -2: set itself in control (for missions where the own sysid is still unknown), -3: remove control if currently in control).| Compid for secondary control (0: no one in control, -1: leave unchanged, -2: set itself in control (for missions where the own sysid is still unknown), -3: remove control if currently in control).| Reserved (default:0)| Reserved (default:0)| Component ID of gimbal device to address (or 1-6 for non-MAVLink gimbal), 0 for all gimbal device components. Send command multiple times for more than one gimbal (but not all gimbals).|  */\n   MAV_CMD_IMAGE_START_CAPTURE=2000, /* Start image capture sequence. CAMERA_IMAGE_CAPTURED must be emitted after each capture.\n\n          Param1 (id) may be used to specify the target camera: 0: all cameras, 1 to 6: autopilot-connected cameras, 7-255: MAVLink camera component ID.\n          It is needed in order to target specific cameras connected to the autopilot, or specific sensors in a multi-sensor camera (neither of which have a distinct MAVLink component ID).\n          It is also needed to specify the target camera in missions.\n\n          When used in a mission, an autopilot should execute the MAV_CMD for a specified local camera (param1 = 1-6), or resend it as a command if it is intended for a MAVLink camera (param1 = 7 - 255), setting the command's target_component as the param1 value (and setting param1 in the command to zero).\n          If the param1 is 0 the autopilot should do both.\n\n          When sent in a command the target MAVLink address is set using target_component.\n          If addressed specifically to an autopilot: param1 should be used in the same way as it is for missions (though command should NACK with MAV_RESULT_DENIED if a specified local camera does not exist).\n          If addressed to a MAVLink camera, param 1 can be used to address all cameras (0), or to separately address 1 to 7 individual sensors. Other values should be NACKed with MAV_RESULT_DENIED.\n          If the command is broadcast (target_component is 0) then param 1 should be set to 0 (any other value should be NACKED with MAV_RESULT_DENIED). An autopilot would trigger any local cameras and forward the command to all channels.\n         |Target camera ID. 7 to 255: MAVLink camera component id. 1 to 6 for cameras that don't have a distinct component id (such as autopilot-attached cameras). 0: all cameras. This is used to specifically target autopilot-connected cameras or individual sensors in a multi-sensor MAVLink camera. It is also used to target specific cameras when the MAV_CMD is used in a mission| Desired elapsed time between two consecutive pictures (in seconds). Minimum values depend on hardware (typically greater than 2 seconds).| Total number of images to capture. 0 to capture forever/until MAV_CMD_IMAGE_STOP_CAPTURE.| Capture sequence number starting from 1. This is only valid for single-capture (param3 == 1), otherwise set to 0. Increment the capture ID for each capture command to prevent double captures when a command is re-transmitted.| Reserved (default:0)| Reserved (default:0)| Reserved (default:NaN)|  */\n   MAV_CMD_IMAGE_STOP_CAPTURE=2001, /* Stop image capture sequence.\n\n          Param1 (id) may be used to specify the target camera: 0: all cameras, 1 to 6: autopilot-connected cameras, 7-255: MAVLink camera component ID.\n          It is needed in order to target specific cameras connected to the autopilot, or specific sensors in a multi-sensor camera (neither of which have a distinct MAVLink component ID).\n          It is also needed to specify the target camera in missions.\n\n          When used in a mission, an autopilot should execute the MAV_CMD for a specified local camera (param1 = 1-6), or resend it as a command if it is intended for a MAVLink camera (param1 = 7 - 255), setting the command's target_component as the param1 value (and setting param1 in the command to zero).\n          If the param1 is 0 the autopilot should do both.\n\n          When sent in a command the target MAVLink address is set using target_component.\n          If addressed specifically to an autopilot: param1 should be used in the same way as it is for missions (though command should NACK with MAV_RESULT_DENIED if a specified local camera does not exist).\n          If addressed to a MAVLink camera, param1 can be used to address all cameras (0), or to separately address 1 to 7 individual sensors. Other values should be NACKed with MAV_RESULT_DENIED.\n          If the command is broadcast (target_component is 0) then param 1 should be set to 0 (any other value should be NACKED with MAV_RESULT_DENIED). An autopilot would trigger any local cameras and forward the command to all channels.\n         |Target camera ID. 7 to 255: MAVLink camera component id. 1 to 6 for cameras that don't have a distinct component id (such as autopilot-attached cameras). 0: all cameras. This is used to specifically target autopilot-connected cameras or individual sensors in a multi-sensor MAVLink camera. It is also used to target specific cameras when the MAV_CMD is used in a mission| Reserved (default:NaN)| Reserved (default:NaN)| Reserved (default:NaN)| Reserved (default:0)| Reserved (default:0)| Reserved (default:NaN)|  */\n   MAV_CMD_REQUEST_CAMERA_IMAGE_CAPTURE=2002, /* Re-request a CAMERA_IMAGE_CAPTURED message. |Sequence number for missing CAMERA_IMAGE_CAPTURED message| Reserved (default:NaN)| Reserved (default:NaN)| Reserved (default:NaN)| Reserved (default:0)| Reserved (default:0)| Reserved (default:NaN)|  */\n   MAV_CMD_DO_TRIGGER_CONTROL=2003, /* Enable or disable on-board camera triggering system. |Trigger enable/disable (0 for disable, 1 for start), -1 to ignore| 1 to reset the trigger sequence, -1 or 0 to ignore| 1 to pause triggering, but without switching the camera off or retracting it. -1 to ignore| Reserved (default:0)| Reserved (default:0)| Reserved (default:0)| Reserved (default:0)|  */\n   MAV_CMD_CAMERA_TRACK_POINT=2004, /* If the camera supports point visual tracking (CAMERA_CAP_FLAGS_HAS_TRACKING_POINT is set), this command allows to initiate the tracking. |Point to track x value (normalized 0..1, 0 is left, 1 is right).| Point to track y value (normalized 0..1, 0 is top, 1 is bottom).| Point radius (normalized 0..1, 0 is one pixel, 1 is full image width).| Reserved (default:0)| Reserved (default:0)| Reserved (default:0)| Reserved (default:0)|  */\n   MAV_CMD_CAMERA_TRACK_RECTANGLE=2005, /* If the camera supports rectangle visual tracking (CAMERA_CAP_FLAGS_HAS_TRACKING_RECTANGLE is set), this command allows to initiate the tracking. |Top left corner of rectangle x value (normalized 0..1, 0 is left, 1 is right).| Top left corner of rectangle y value (normalized 0..1, 0 is top, 1 is bottom).| Bottom right corner of rectangle x value (normalized 0..1, 0 is left, 1 is right).| Bottom right corner of rectangle y value (normalized 0..1, 0 is top, 1 is bottom).| Reserved (default:0)| Reserved (default:0)| Reserved (default:0)|  */\n   MAV_CMD_CAMERA_STOP_TRACKING=2010, /* Stops ongoing tracking. |Reserved (default:0)| Reserved (default:0)| Reserved (default:0)| Reserved (default:0)| Reserved (default:0)| Reserved (default:0)| Reserved (default:0)|  */\n   MAV_CMD_VIDEO_START_CAPTURE=2500, /* Starts video capture (recording). |Video Stream ID (0 for all streams)| Frequency CAMERA_CAPTURE_STATUS messages should be sent while recording (0 for no messages, otherwise frequency)| Reserved (default:NaN)| Reserved (default:NaN)| Reserved (default:0)| Reserved (default:0)| Reserved (default:NaN)|  */\n   MAV_CMD_VIDEO_STOP_CAPTURE=2501, /* Stop the current video capture (recording). |Video Stream ID (0 for all streams)| Reserved (default:NaN)| Reserved (default:NaN)| Reserved (default:NaN)| Reserved (default:0)| Reserved (default:0)| Reserved (default:NaN)|  */\n   MAV_CMD_VIDEO_START_STREAMING=2502, /* Start video streaming |Video Stream ID (0 for all streams, 1 for first, 2 for second, etc.)| Reserved (default:0)| Reserved (default:0)| Reserved (default:0)| Reserved (default:0)| Reserved (default:0)| Reserved (default:0)|  */\n   MAV_CMD_VIDEO_STOP_STREAMING=2503, /* Stop the given video stream |Video Stream ID (0 for all streams, 1 for first, 2 for second, etc.)| Reserved (default:0)| Reserved (default:0)| Reserved (default:0)| Reserved (default:0)| Reserved (default:0)| Reserved (default:0)|  */\n   MAV_CMD_REQUEST_VIDEO_STREAM_INFORMATION=2504, /* Request video stream information (VIDEO_STREAM_INFORMATION) |Video Stream ID (0 for all streams, 1 for first, 2 for second, etc.)| Reserved (default:0)| Reserved (default:0)| Reserved (default:0)| Reserved (default:0)| Reserved (default:0)| Reserved (default:0)|  */\n   MAV_CMD_REQUEST_VIDEO_STREAM_STATUS=2505, /* Request video stream status (VIDEO_STREAM_STATUS) |Video Stream ID (0 for all streams, 1 for first, 2 for second, etc.)| Reserved (default:0)| Reserved (default:0)| Reserved (default:0)| Reserved (default:0)| Reserved (default:0)| Reserved (default:0)|  */\n   MAV_CMD_LOGGING_START=2510, /* Request to start streaming logging data over MAVLink (see also LOGGING_DATA message) |Format: 0: ULog| Reserved (set to 0)| Reserved (set to 0)| Reserved (set to 0)| Reserved (set to 0)| Reserved (set to 0)| Reserved (set to 0)|  */\n   MAV_CMD_LOGGING_STOP=2511, /* Request to stop streaming log data over MAVLink |Reserved (set to 0)| Reserved (set to 0)| Reserved (set to 0)| Reserved (set to 0)| Reserved (set to 0)| Reserved (set to 0)| Reserved (set to 0)|  */\n   MAV_CMD_AIRFRAME_CONFIGURATION=2520, /*  |Landing gear ID (default: 0, -1 for all)| Landing gear position (Down: 0, Up: 1, NaN for no change)| Reserved (default:NaN)| Reserved (default:NaN)| Reserved (default:0)| Reserved (default:0)| Reserved (default:NaN)|  */\n   MAV_CMD_CONTROL_HIGH_LATENCY=2600, /* Request to start/stop transmitting over the high latency telemetry |Control transmission over high latency telemetry (0: stop, 1: start)| Empty| Empty| Empty| Empty| Empty| Empty|  */\n   MAV_CMD_PANORAMA_CREATE=2800, /* Create a panorama at the current position |Viewing angle horizontal of the panorama (+- 0.5 the total angle)| Viewing angle vertical of panorama.| Speed of the horizontal rotation.| Speed of the vertical rotation.| Reserved (default:0)| Reserved (default:0)| Reserved (default:0)|  */\n   MAV_CMD_DO_VTOL_TRANSITION=3000, /* Request VTOL transition |The target VTOL state. For normal transitions, only MAV_VTOL_STATE_MC and MAV_VTOL_STATE_FW can be used.| Force immediate transition to the specified MAV_VTOL_STATE. 1: Force immediate, 0: normal transition. Can be used, for example, to trigger an emergency \"Quadchute\". Caution: Can be dangerous/damage vehicle, depending on autopilot implementation of this command.| Reserved (default:0)| Reserved (default:0)| Reserved (default:0)| Reserved (default:0)| Reserved (default:0)|  */\n   MAV_CMD_ARM_AUTHORIZATION_REQUEST=3001, /* Request authorization to arm the vehicle to a external entity, the arm authorizer is responsible to request all data that is needs from the vehicle before authorize or deny the request.\n\t\tIf approved the COMMAND_ACK message progress field should be set with period of time that this authorization is valid in seconds.\n\t\tIf the authorization is denied COMMAND_ACK.result_param2 should be set with one of the reasons in ARM_AUTH_DENIED_REASON.\n         |Vehicle system id, this way ground station can request arm authorization on behalf of any vehicle| Reserved (default:0)| Reserved (default:0)| Reserved (default:0)| Reserved (default:0)| Reserved (default:0)| Reserved (default:0)|  */\n   MAV_CMD_SET_GUIDED_SUBMODE_STANDARD=4000, /* This command sets the submode to standard guided when vehicle is in guided mode. The vehicle holds position and altitude and the user can input the desired velocities along all three axes.\n                   |Reserved (default:0)| Reserved (default:0)| Reserved (default:0)| Reserved (default:0)| Reserved (default:0)| Reserved (default:0)| Reserved (default:0)|  */\n   MAV_CMD_SET_GUIDED_SUBMODE_CIRCLE=4001, /* This command sets submode circle when vehicle is in guided mode. Vehicle flies along a circle facing the center of the circle. The user can input the velocity along the circle and change the radius. If no input is given the vehicle will hold position.\n                   |Radius of desired circle in CIRCLE_MODE| User defined| User defined| User defined| Target latitude of center of circle in CIRCLE_MODE| Target longitude of center of circle in CIRCLE_MODE| Reserved (default:0)|  */\n   MAV_CMD_CONDITION_GATE=4501, /* Delay mission state machine until gate has been reached. |Geometry: 0: orthogonal to path between previous and next waypoint.| Altitude: 0: ignore altitude| Empty| Empty| Latitude| Longitude| Altitude|  */\n   MAV_CMD_NAV_FENCE_RETURN_POINT=5000, /* Fence return point (there can only be one such point in a geofence definition). If rally points are supported they should be used instead. |Reserved| Reserved| Reserved| Reserved| Latitude| Longitude| Altitude|  */\n   MAV_CMD_NAV_FENCE_POLYGON_VERTEX_INCLUSION=5001, /* Fence vertex for an inclusion polygon (the polygon must not be self-intersecting). The vehicle must stay within this area. Minimum of 3 vertices required.\n         |Polygon vertex count| Vehicle must be inside ALL inclusion zones in a single group, vehicle must be inside at least one group, must be the same for all points in each polygon| Reserved| Reserved| Latitude| Longitude| Reserved|  */\n   MAV_CMD_NAV_FENCE_POLYGON_VERTEX_EXCLUSION=5002, /* Fence vertex for an exclusion polygon (the polygon must not be self-intersecting). The vehicle must stay outside this area. Minimum of 3 vertices required.\n         |Polygon vertex count| Reserved| Reserved| Reserved| Latitude| Longitude| Reserved|  */\n   MAV_CMD_NAV_FENCE_CIRCLE_INCLUSION=5003, /* Circular fence area. The vehicle must stay inside this area.\n         |Radius.| Vehicle must be inside ALL inclusion zones in a single group, vehicle must be inside at least one group| Reserved| Reserved| Latitude| Longitude| Reserved|  */\n   MAV_CMD_NAV_FENCE_CIRCLE_EXCLUSION=5004, /* Circular fence area. The vehicle must stay outside this area.\n         |Radius.| Reserved| Reserved| Reserved| Latitude| Longitude| Reserved|  */\n   MAV_CMD_NAV_RALLY_POINT=5100, /* Rally point. You can have multiple rally points defined.\n         |Reserved| Reserved| Reserved| Reserved| Latitude| Longitude| Altitude|  */\n   MAV_CMD_UAVCAN_GET_NODE_INFO=5200, /* Commands the vehicle to respond with a sequence of messages UAVCAN_NODE_INFO, one message per every UAVCAN node that is online. Note that some of the response messages can be lost, which the receiver can detect easily by checking whether every received UAVCAN_NODE_STATUS has a matching message UAVCAN_NODE_INFO received earlier; if not, this command should be sent again in order to request re-transmission of the node information messages. |Reserved (set to 0)| Reserved (set to 0)| Reserved (set to 0)| Reserved (set to 0)| Reserved (set to 0)| Reserved (set to 0)| Reserved (set to 0)|  */\n   MAV_CMD_DO_SET_SAFETY_SWITCH_STATE=5300, /* Change state of safety switch. |New safety switch state.| Empty.| Empty.| Empty| Empty.| Empty.| Empty.|  */\n   MAV_CMD_DO_ADSB_OUT_IDENT=10001, /* Trigger the start of an ADSB-out IDENT. This should only be used when requested to do so by an Air Traffic Controller in controlled airspace. This starts the IDENT which is then typically held for 18 seconds by the hardware per the Mode A, C, and S transponder spec. |Reserved (set to 0)| Reserved (set to 0)| Reserved (set to 0)| Reserved (set to 0)| Reserved (set to 0)| Reserved (set to 0)| Reserved (set to 0)|  */\n   MAV_CMD_PAYLOAD_PREPARE_DEPLOY=30001, /* Deploy payload on a Lat / Lon / Alt position. This includes the navigation to reach the required release position and velocity. |Operation mode. 0: prepare single payload deploy (overwriting previous requests), but do not execute it. 1: execute payload deploy immediately (rejecting further deploy commands during execution, but allowing abort). 2: add payload deploy to existing deployment list.| Desired approach vector in compass heading. A negative value indicates the system can define the approach vector at will.| Desired ground speed at release time. This can be overridden by the airframe in case it needs to meet minimum airspeed. A negative value indicates the system can define the ground speed at will.| Minimum altitude clearance to the release position. A negative value indicates the system can define the clearance at will.| Latitude.| Longitude.| Altitude (MSL)|  */\n   MAV_CMD_PAYLOAD_CONTROL_DEPLOY=30002, /* Control the payload deployment. |Operation mode. 0: Abort deployment, continue normal mission. 1: switch to payload deployment mode. 100: delete first payload deployment request. 101: delete all payload deployment requests.| Reserved| Reserved| Reserved| Reserved| Reserved| Reserved|  */\n   MAV_CMD_WAYPOINT_USER_1=31000, /* User defined waypoint item. Ground Station will show the Vehicle as flying through this item. |User defined| User defined| User defined| User defined| Latitude unscaled| Longitude unscaled| Altitude (MSL)|  */\n   MAV_CMD_WAYPOINT_USER_2=31001, /* User defined waypoint item. Ground Station will show the Vehicle as flying through this item. |User defined| User defined| User defined| User defined| Latitude unscaled| Longitude unscaled| Altitude (MSL)|  */\n   MAV_CMD_WAYPOINT_USER_3=31002, /* User defined waypoint item. Ground Station will show the Vehicle as flying through this item. |User defined| User defined| User defined| User defined| Latitude unscaled| Longitude unscaled| Altitude (MSL)|  */\n   MAV_CMD_WAYPOINT_USER_4=31003, /* User defined waypoint item. Ground Station will show the Vehicle as flying through this item. |User defined| User defined| User defined| User defined| Latitude unscaled| Longitude unscaled| Altitude (MSL)|  */\n   MAV_CMD_WAYPOINT_USER_5=31004, /* User defined waypoint item. Ground Station will show the Vehicle as flying through this item. |User defined| User defined| User defined| User defined| Latitude unscaled| Longitude unscaled| Altitude (MSL)|  */\n   MAV_CMD_SPATIAL_USER_1=31005, /* User defined spatial item. Ground Station will not show the Vehicle as flying through this item. Example: ROI item. |User defined| User defined| User defined| User defined| Latitude unscaled| Longitude unscaled| Altitude (MSL)|  */\n   MAV_CMD_SPATIAL_USER_2=31006, /* User defined spatial item. Ground Station will not show the Vehicle as flying through this item. Example: ROI item. |User defined| User defined| User defined| User defined| Latitude unscaled| Longitude unscaled| Altitude (MSL)|  */\n   MAV_CMD_SPATIAL_USER_3=31007, /* User defined spatial item. Ground Station will not show the Vehicle as flying through this item. Example: ROI item. |User defined| User defined| User defined| User defined| Latitude unscaled| Longitude unscaled| Altitude (MSL)|  */\n   MAV_CMD_SPATIAL_USER_4=31008, /* User defined spatial item. Ground Station will not show the Vehicle as flying through this item. Example: ROI item. |User defined| User defined| User defined| User defined| Latitude unscaled| Longitude unscaled| Altitude (MSL)|  */\n   MAV_CMD_SPATIAL_USER_5=31009, /* User defined spatial item. Ground Station will not show the Vehicle as flying through this item. Example: ROI item. |User defined| User defined| User defined| User defined| Latitude unscaled| Longitude unscaled| Altitude (MSL)|  */\n   MAV_CMD_USER_1=31010, /* User defined command. Ground Station will not show the Vehicle as flying through this item. Example: MAV_CMD_DO_SET_PARAMETER item. |User defined| User defined| User defined| User defined| User defined| User defined| User defined|  */\n   MAV_CMD_USER_2=31011, /* User defined command. Ground Station will not show the Vehicle as flying through this item. Example: MAV_CMD_DO_SET_PARAMETER item. |User defined| User defined| User defined| User defined| User defined| User defined| User defined|  */\n   MAV_CMD_USER_3=31012, /* User defined command. Ground Station will not show the Vehicle as flying through this item. Example: MAV_CMD_DO_SET_PARAMETER item. |User defined| User defined| User defined| User defined| User defined| User defined| User defined|  */\n   MAV_CMD_USER_4=31013, /* User defined command. Ground Station will not show the Vehicle as flying through this item. Example: MAV_CMD_DO_SET_PARAMETER item. |User defined| User defined| User defined| User defined| User defined| User defined| User defined|  */\n   MAV_CMD_USER_5=31014, /* User defined command. Ground Station will not show the Vehicle as flying through this item. Example: MAV_CMD_DO_SET_PARAMETER item. |User defined| User defined| User defined| User defined| User defined| User defined| User defined|  */\n   MAV_CMD_CAN_FORWARD=32000, /* Request forwarding of CAN packets from the given CAN bus to this component. CAN Frames are sent using CAN_FRAME and CANFD_FRAME messages |Bus number (0 to disable forwarding, 1 for first bus, 2 for 2nd bus, 3 for 3rd bus).| Empty.| Empty.| Empty.| Empty.| Empty.| Empty.|  */\n   MAV_CMD_FIXED_MAG_CAL_YAW=42006, /* Magnetometer calibration based on provided known yaw. This allows for fast calibration using WMM field tables in the vehicle, given only the known yaw of the vehicle. If Latitude and longitude are both zero then use the current vehicle location. |Yaw of vehicle in earth frame.| CompassMask, 0 for all.| Latitude.| Longitude.| Empty.| Empty.| Empty.|  */\n   MAV_CMD_DO_WINCH=42600, /* Command to operate winch. |Winch instance number.| Action to perform.| Length of line to release (negative to wind).| Release rate (negative to wind).| Empty.| Empty.| Empty.|  */\n   MAV_CMD_EXTERNAL_POSITION_ESTIMATE=43003, /* Provide an external position estimate for use when dead-reckoning. This is meant to be used for occasional position resets that may be provided by a external system such as a remote pilot using landmarks over a video link. |Timestamp that this message was sent as a time in the transmitters time domain. The sender should wrap this time back to zero based on required timing accuracy for the application and the limitations of a 32 bit float. For example, wrapping at 10 hours would give approximately 1ms accuracy. Recipient must handle time wrap in any timing jitter correction applied to this field. Wrap rollover time should not be at not more than 250 seconds, which would give approximately 10 microsecond accuracy.| The time spent in processing the sensor data that is the basis for this position. The recipient can use this to improve time alignment of the data. Set to zero if not known.| estimated one standard deviation accuracy of the measurement. Set to NaN if not known.| Empty| Latitude| Longitude| Altitude, not used. Should be sent as NaN. May be supported in a future version of this message.|  */\n   MAV_CMD_ENUM_END=43004, /*  | */"
  n1 = Unbundle By Name("COMMAND_LONG") -> ("self"=w46:cluster{"system_id":u8, "component_id":u8}, "target_system"=w4:u8, "target_component"=w3:u8, "command (MAV_CMD)"=w6:u16, "confirmation"=w2:u8, "param1"=w34:sgl, "param2"=w26:sgl, "param3"=w19:sgl, "param4"=w18:sgl, "param5"=w17:sgl, "param6"=w13:sgl, "param7"=w10:sgl)
  n2 = Unbundle(w46) -> ("system_id"=w40:u8, "component_id"=w39:u8)
  n3 = Type Cast(type=u8[] [] ("index"), x=w34) -> (*(type *) &x=w35:u8[])
  n4 = Type Cast(type=u8[] [] ("index"), x=w26) -> (*(type *) &x=w31:u8[])
  n5 = Type Cast(type=u8[] [] ("index"), x=w19) -> (*(type *) &x=w29:u8[])
  n6 = Type Cast(type=u8[] [] ("index"), x=w18) -> (*(type *) &x=w27:u8[])
  n7 = Type Cast(type=u8[] [] ("index"), x=w17) -> (*(type *) &x=w21:u8[])
  n8 = Type Cast(type=u8[] [] ("index"), x=w13) -> (*(type *) &x=w15:u8[])
  n9 = Type Cast(type=u8[] [] ("index"), x=w10) -> (*(type *) &x=w11:u8[])
  n10 = Type Cast(type=u8[] [] ("index"), x=w6) -> (*(type *) &x=w7:u8[])
  n11 = Reverse 1D Array(array=w35) -> (reversed array=w33:u8[])
  n12 = Reverse 1D Array(array=w31) -> (reversed array=w25:u8[])
  n13 = Reverse 1D Array(array=w29) -> (reversed array=w24:u8[])
  n14 = Reverse 1D Array(array=w27) -> (reversed array=w23:u8[])
  n15 = Reverse 1D Array(array=w21) -> (reversed array=w20:u8[])
  n16 = Reverse 1D Array(array=w15) -> (reversed array=w14:u8[])
  n17 = Reverse 1D Array(array=w11) -> (reversed array=w9:u8[])
  n18 = Reverse 1D Array(array=w7) -> (reversed array=w5:u8[])
  n19 = Insert Into Array(array=u8[] [33, 0, 0, 255, 255, 255, 76, 0, 0], new element #1=w33, new element #2=w25, new element #3=w24, new element #4=w23, new element #5=w20, new element #6=w14, new element #7=w9, new element #8=w5, new element #9=w4, new element #10=w3, new element #11=w2) -> (w37:u8[])  [unwired: 1 in]
  n20 = Increment(x="packet_sequence_in") -> (x+1=→"packet_sequence_out":u8)
  n21 = Replace Array Subset(array=w37, new element #1="packet_sequence_in", index #1=3 ("index"), new element #2=w40, index #2=4 ("index"), new element #3=w39, index #3=5 ("index")) -> (w38:u8[])
  n22 = call "mav_crc_send.vi"("Byte In"=w38) -> ("Output Byte"=→"mavlink_buffer_out":u8[])  [unwired: 10 in]
